vi "Get RemIO Library Path.vi"(11 "name or relative path":string) -> (3 "appended path":path)   [LabVIEW 2017, in "Modules.lvlib"]
uses:
  Modules.lvlib
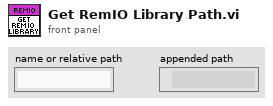
[diagram p1: front panel]
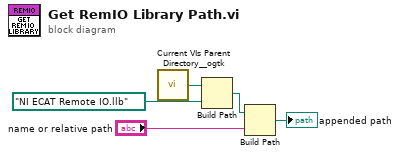
[diagram p0: block diagram]
diagram:
  n1 = call <userlib>:"Current VIs Parent Directory__ogtk.vi"() -> ("Parent Directory (+ Relative)"=w2:path)  [unwired: 5 in]
  n2 = Build Path(base path=w2, name or relative path=path "NI ECAT Remote IO.llb" ("vi path")) -> (appended path=w3:path)
  n3 = Build Path(base path=w3, name or relative path="name or relative path") -> (appended path=→"appended path":path)
